vi "HW_6p1_Task2_fishele.vi"() -> ()   [LabVIEW 2021]
panel:
  out "Number of times Temp > 250C (Valve opens)":dbl
  out "Average Temp":dbl
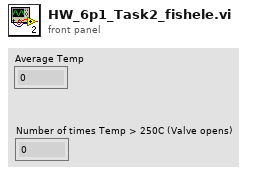
[diagram p1: front panel]
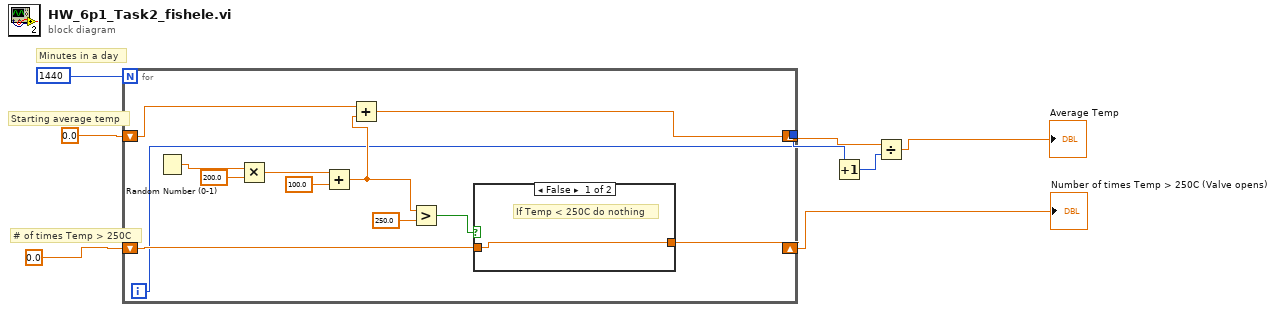
[diagram p0: block diagram]
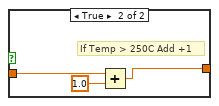
[diagram p2: hidden frame]
diagram:
  # "# of times Temp > 250C"
  # "Starting average temp"
  # "Minutes in a day"
  n1 = for {
    N: 1440 -> [_]
    shift-right: [w14] -> w6
    shift-left: 0.0 -> [w13]
    shift-right: [w11] -> w3
    shift-left: 0.0 -> [w10]
    tunnel: [w9] -> w4
    i -> [w9]
    n2 = Random Number (0-1)() -> (number: 0 to 1=w20:dbl)
    n3 = Multiply(x=w20, y=200.0) -> (x*y=w18:dbl)
    n4 = Add(x=w18, y=100.0) -> (x+y=w12:dbl)
    n5 = Add(x=w10, y=w12) -> (x+y=w11:dbl)
    n6 = Greater?(x=w12, y=250.0) -> (0:w15:bool)
    n7 = case shown="False" w15 {
      tunnel: w13 -> [w21 w24]
      tunnel: [w21 w22] -> w14
      frame False {
        # "If Temp < 250C do nothing"
      }
      frame True {
        # "If Temp > 250C Add +1"
        n8 = Add(x=w24, y=1.0) -> (x+y=w22:dbl)
      }
    }
  }
  "Number of times Temp > 250C (Valve opens)" <- w6
  n9 = Increment(x=w4) -> (x+1=w2:i32)
  n10 = Divide(x=w3, y=w2) -> (x/y=→"Average Temp":dbl)
